vi "总磷总氮测量数据储存.vi"   [LabVIEW 2016, in "斯坦道总磷总氮V2.lvlib"]
types:
  T1 = cluster{"时间标识":timestamp, "测量模式":enum16{"维护数据", "水样测试", "标样核查", "零点核查", "跨度核查", "空白测试", "平行样测试", "加标回收", "空白校准", "标样校准", "初始化（清洗）", "快捷测试"}, "数据标记表":string, "监测值":sgl, "单位":u16, "数据标识":string, "因子编码":u32, "标样参考值":sgl, "F0":sgl, "F1":sgl, "F2":sgl, "F3":sgl, "F4":sgl, "F5":sgl, "F6":sgl, "F7":sgl, "X":sgl, "温度":sgl, "湿度":sgl, "量程标识":string, "SN":string, "跨度值":sgl, "X1":sgl}
  T2 = enum16{"维护数据", "水样测试", "标样核查", "零点核查", "跨度核查", "空白测试", "平行样测试", "加标回收", "空白校准", "标样校准", "初始化（清洗）", "快捷测试"}
  T3 = enum16{"维护数据", "水样测试", "标样核查", "零点核查", "跨度核查", "空白测试", "平行样测试", "加标回收", "空白校准", "标样校准", "初始化（清洗）"}
  T4 = cluster{"系统时间":timestamp, "工作状态":u16, "测量模式":enum16{"待机", "连续模式", "周期模式", "定点模式", "受控模式", "手动模式"}, "告警代码":u16, "故障代码":u16, "日志代码":u16, "软件版本":u16, "F0":sgl, "F1":sgl, "F2":sgl, "F3":sgl, "T":sgl, "H":sgl, "id":u16, "flowid":u16, "量程":u16, "总磷控温温度1":sgl, "营养盐控温温度2":sgl, "ADC":sgl}
  T5 = cluster{"运行模式":enum16{"维护模式", "常规模式", "应急模式", "质控模式"}, "质控频次":enum16{"关闭", "每天", "星期一", "星期二", "星期三", "星期四", "星期五", "星期六", "星期日"}, "空白核查时间":u16, "跨度核查时间":u16, "测量间隔":dbl}
  T6 = cluster{"因子编码":u32, "单位":u16, "标样参考值":sgl, "水样数据时间":timestamp, "水样实测值":sgl, "水样数据标识":string, "标样数据时间":timestamp, "标样实测值":sgl, "标样数据标识":string, "空白数据时间":timestamp, "空白实测值":sgl, "空白数据标识":string, "零点核查数据时间":timestamp, "零点核查实测值":sgl, "零点核查数据标识":string, "跨度核查数据时间":timestamp, "跨度核查实测值":sgl, "跨度核查数据标识":string, "加标回收数据时间":timestamp, "加标回收实测值":sgl, "加标回收数据标识":string, "平行样数据时间":timestamp, "平行样实测值":sgl, "平行样数据标识":string, "F0":sgl, "F1":sgl, "F2":sgl, "F3":sgl, "F4":sgl, "F5":sgl, "F6":sgl, "F7":sgl, "温度":sgl, "湿度":sgl, "X值":sgl, "fidrange":u16}[]
  T7 = cluster{"因子编码":u32, "单位":u16, "标样参考值":sgl, "水样数据时间":timestamp, "水样实测值":sgl, "水样数据标识":string, "标样数据时间":timestamp, "标样实测值":sgl, "标样数据标识":string, "空白数据时间":timestamp, "空白实测值":sgl, "空白数据标识":string, "零点核查数据时间":timestamp, "零点核查实测值":sgl, "零点核查数据标识":string, "跨度核查数据时间":timestamp, "跨度核查实测值":sgl, "跨度核查数据标识":string, "加标回收数据时间":timestamp, "加标回收实测值":sgl, "加标回收数据标识":string, "平行样数据时间":timestamp, "平行样实测值":sgl, "平行样数据标识":string, "F0":sgl, "F1":sgl, "F2":sgl, "F3":sgl, "F4":sgl, "F5":sgl, "F6":sgl, "F7":sgl, "温度":sgl, "湿度":sgl, "X值":sgl, "fidrange":u16}
  T8 = cluster{"总磷跨度值":dbl, "总磷零点标准液浓度":dbl, "总磷跨度标准液浓度":dbl, "总磷标准液标准浓度":dbl, "总氮跨度值":dbl, "总氮零点标准液浓度":dbl, "总氮跨度标准液浓度":dbl, "总氮标准液标准浓度":dbl, "COD跨度值":dbl, "COD零点标准液浓度":dbl, "COD跨度标准液浓度":dbl, "COD标准液标准浓度":dbl, "氨氮跨度值":dbl, "氨氮零点标准液浓度":dbl, "氨氮跨度标准液浓度":dbl, "氨氮标准液标准浓度":dbl, "磷酸盐跨度值":dbl, "磷酸盐零点标准液浓度":dbl, "磷酸盐跨度标准液浓度":dbl, "磷酸盐标准液标准浓度":dbl, "硝氮跨度值":dbl, "硝氮零点标准液浓度":dbl, "硝氮跨度标准液浓度":dbl, "硝氮标准液标准浓度":dbl, "亚硝氮跨度值":dbl, "亚硝氮零点标准液浓度":dbl, "亚硝氮跨度标准液浓度":dbl, "亚硝氮标准液标准浓度":dbl, "硫化物跨度值":dbl, "硫化物零点标准液浓度":dbl, "硫化物跨度标准液浓度":dbl, "硫化物标准液标准浓度":dbl, "硅酸盐跨度值":dbl, "硅酸盐零点标准液浓度":dbl, "硅酸盐跨度标准液浓度":dbl, "硅酸盐标准液标准浓度":dbl}
  T9 = typedef "斯坦道总磷总氮V2.lvlib/关键参数.ctl" = cluster{"测量量程":sgl, "测量检出限":sgl, "测量精度":sgl, "测量间隔":sgl, "消解温度":sgl, "消解时长":sgl, "三项式系数":sgl, "二次多项式系数":sgl, "曲线斜率":sgl, "曲线截距":sgl, "线性相关系数":sgl, "空白校准时间":timestamp, "标样校准时间":timestamp, "测量信号值":sgl, "稀释倍数":sgl, "空白标定系数":sgl, "量程系数":sgl}
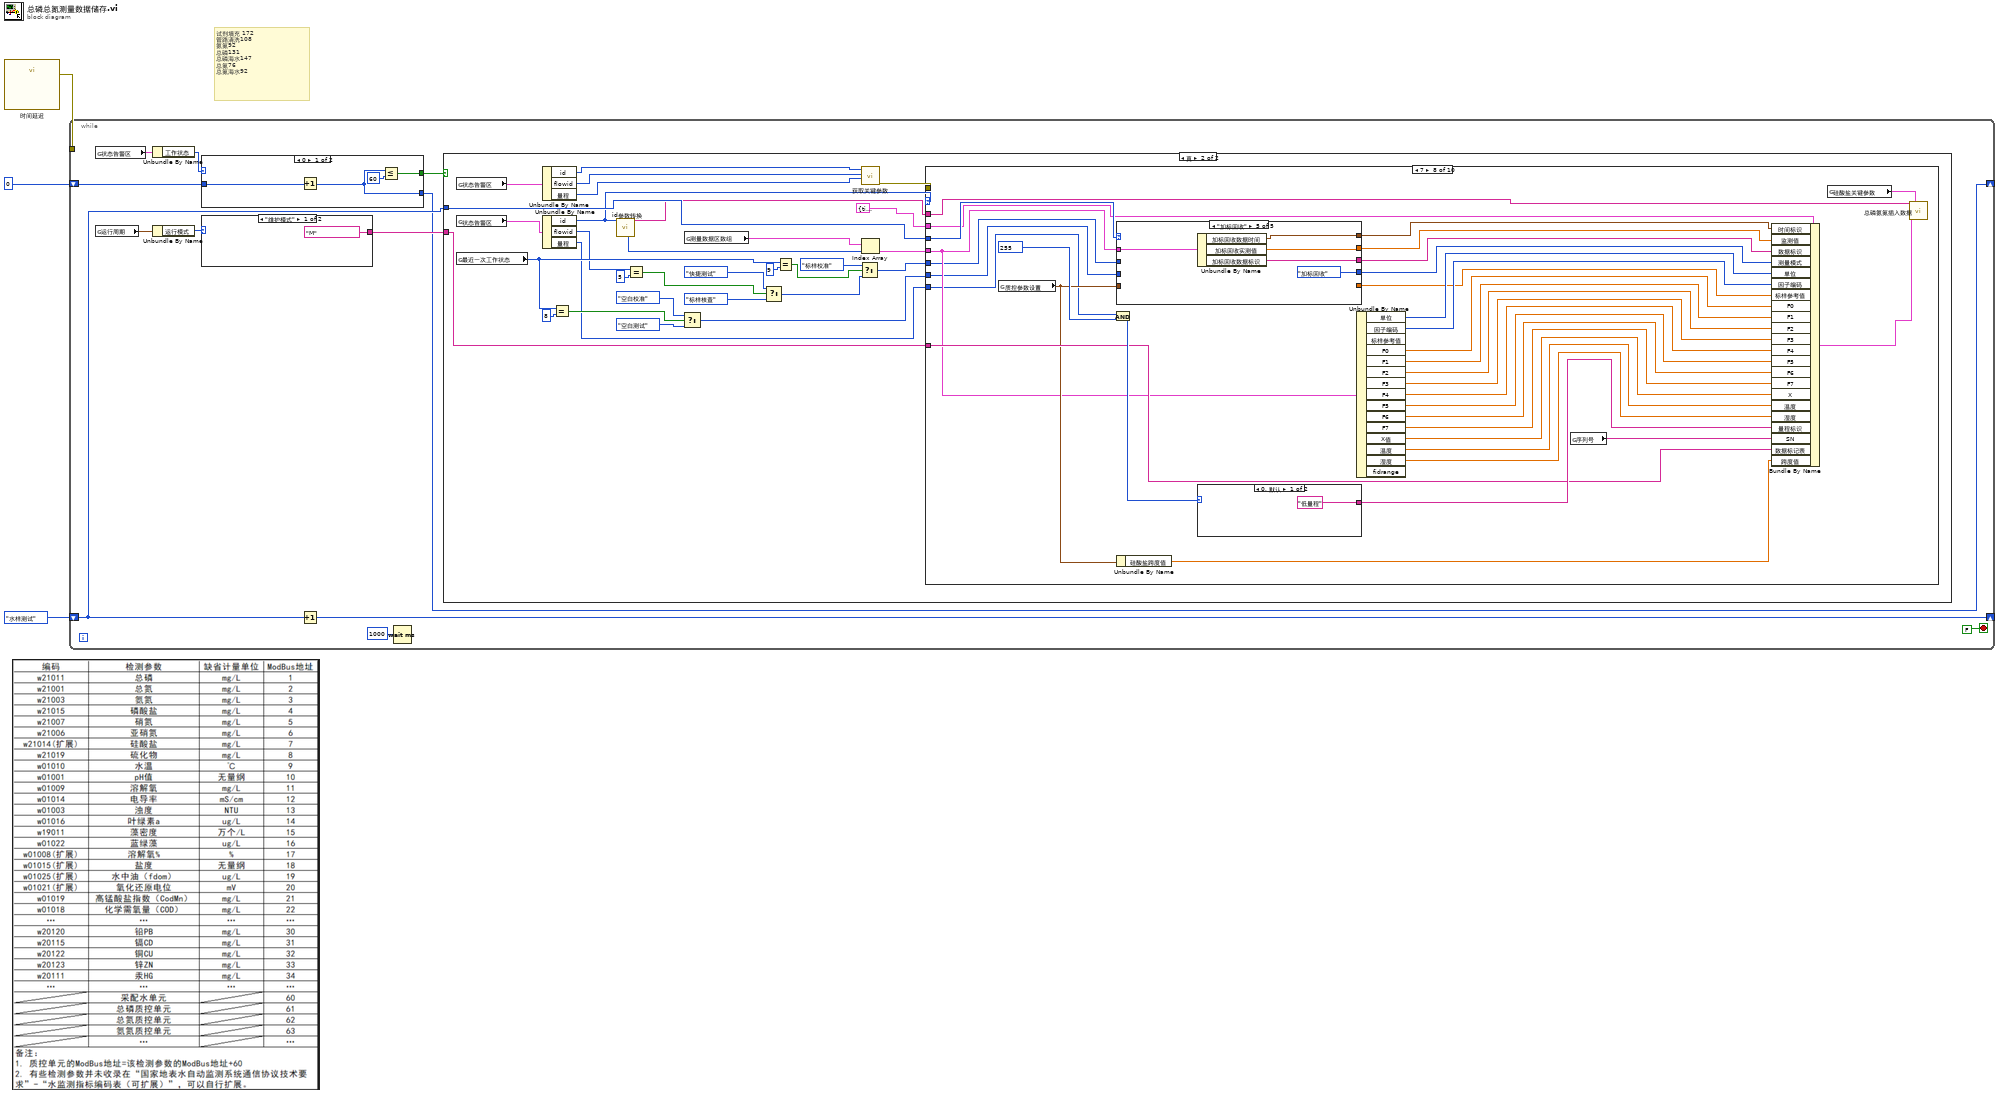
[diagram p0: block diagram]
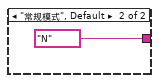
[diagram p3: hidden frame]
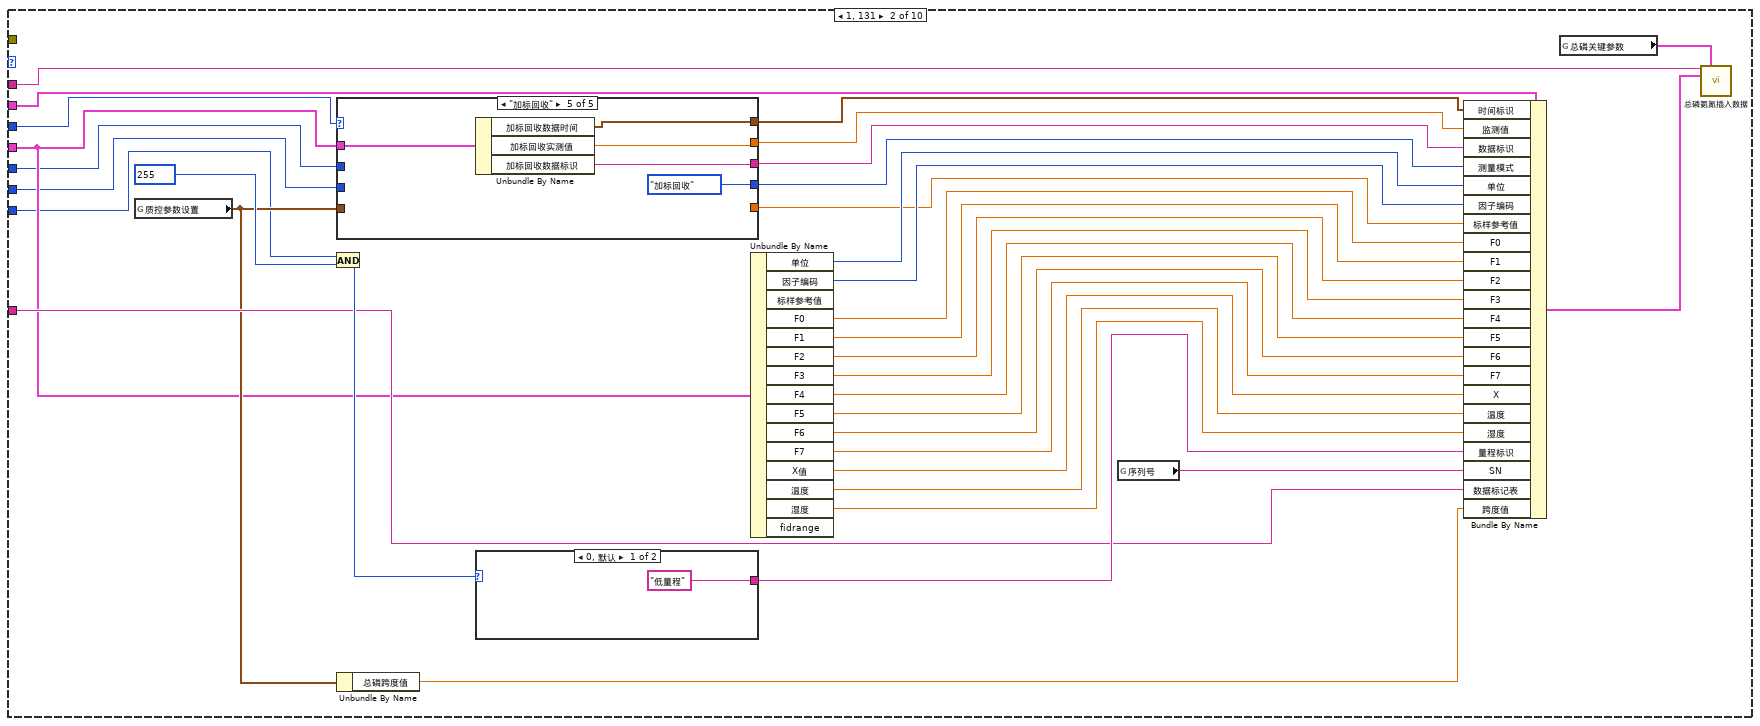
[diagram p6: hidden frame]
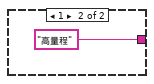
[diagram p7: hidden frame]
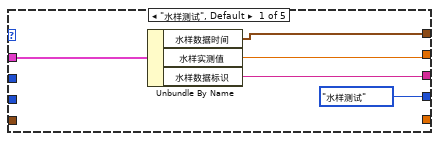
[diagram p8: hidden frame]
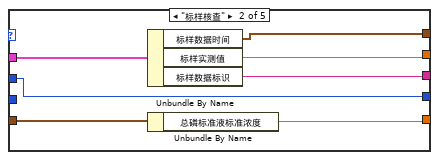
[diagram p9: hidden frame]
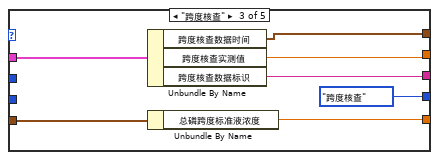
[diagram p10: hidden frame]
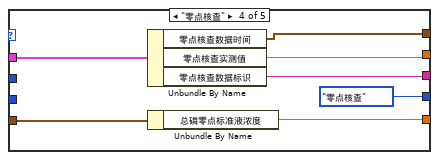
[diagram p11: hidden frame]
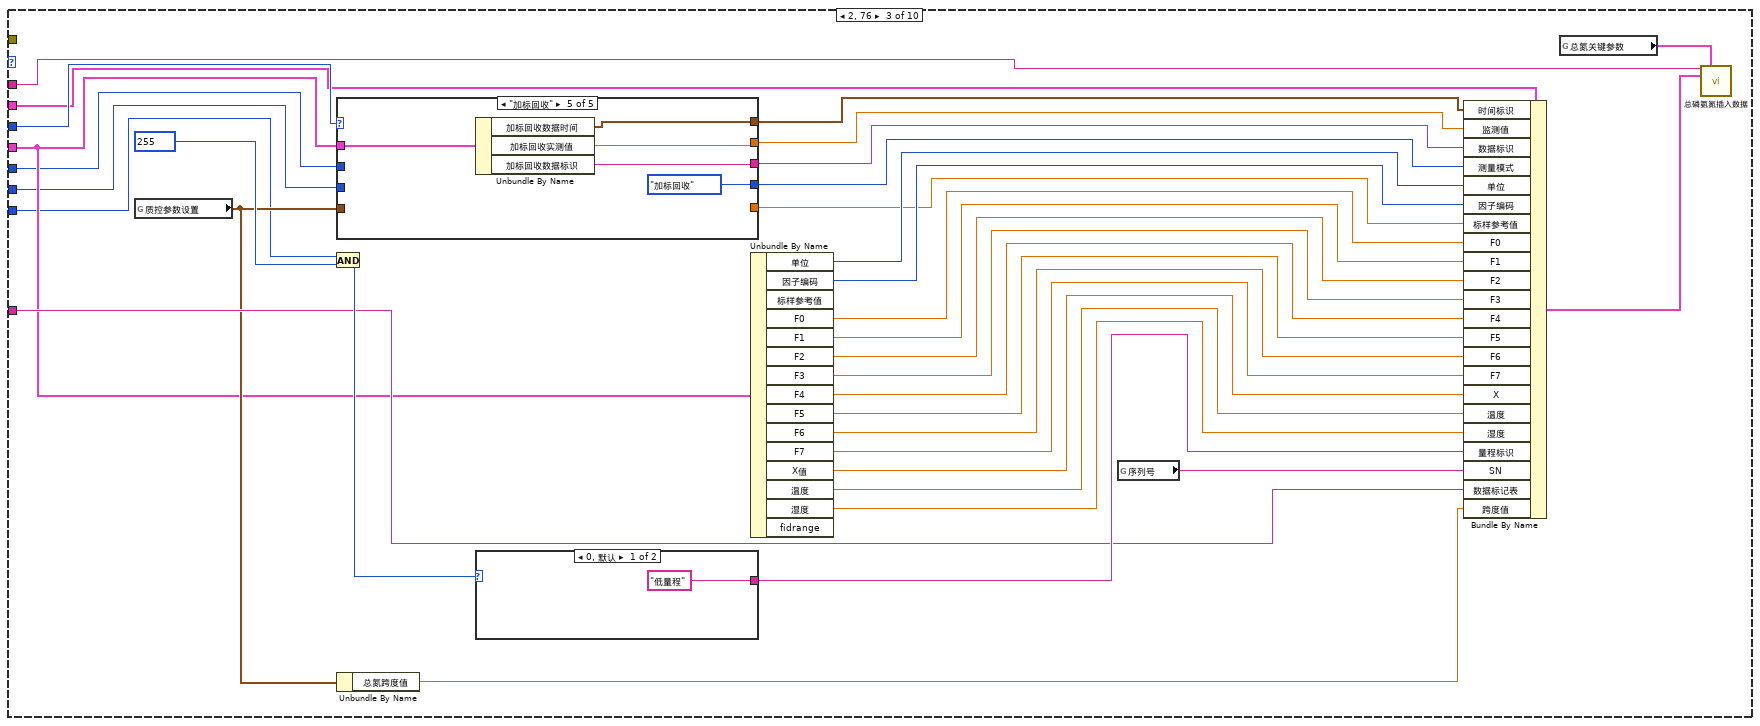
[diagram p12: hidden frame]
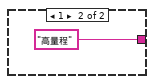
[diagram p13: hidden frame]
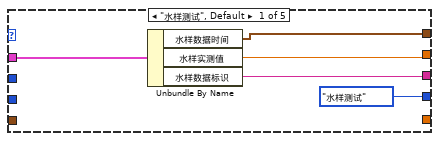
[diagram p14: hidden frame]
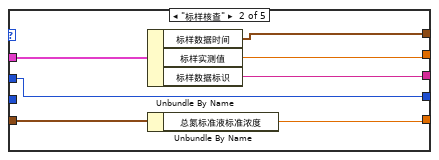
[diagram p15: hidden frame]
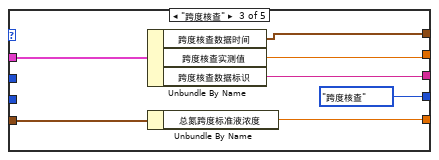
[diagram p16: hidden frame]
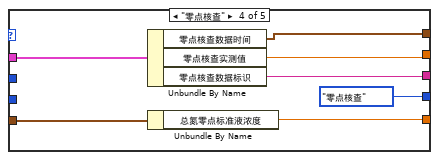
[diagram p17: hidden frame]
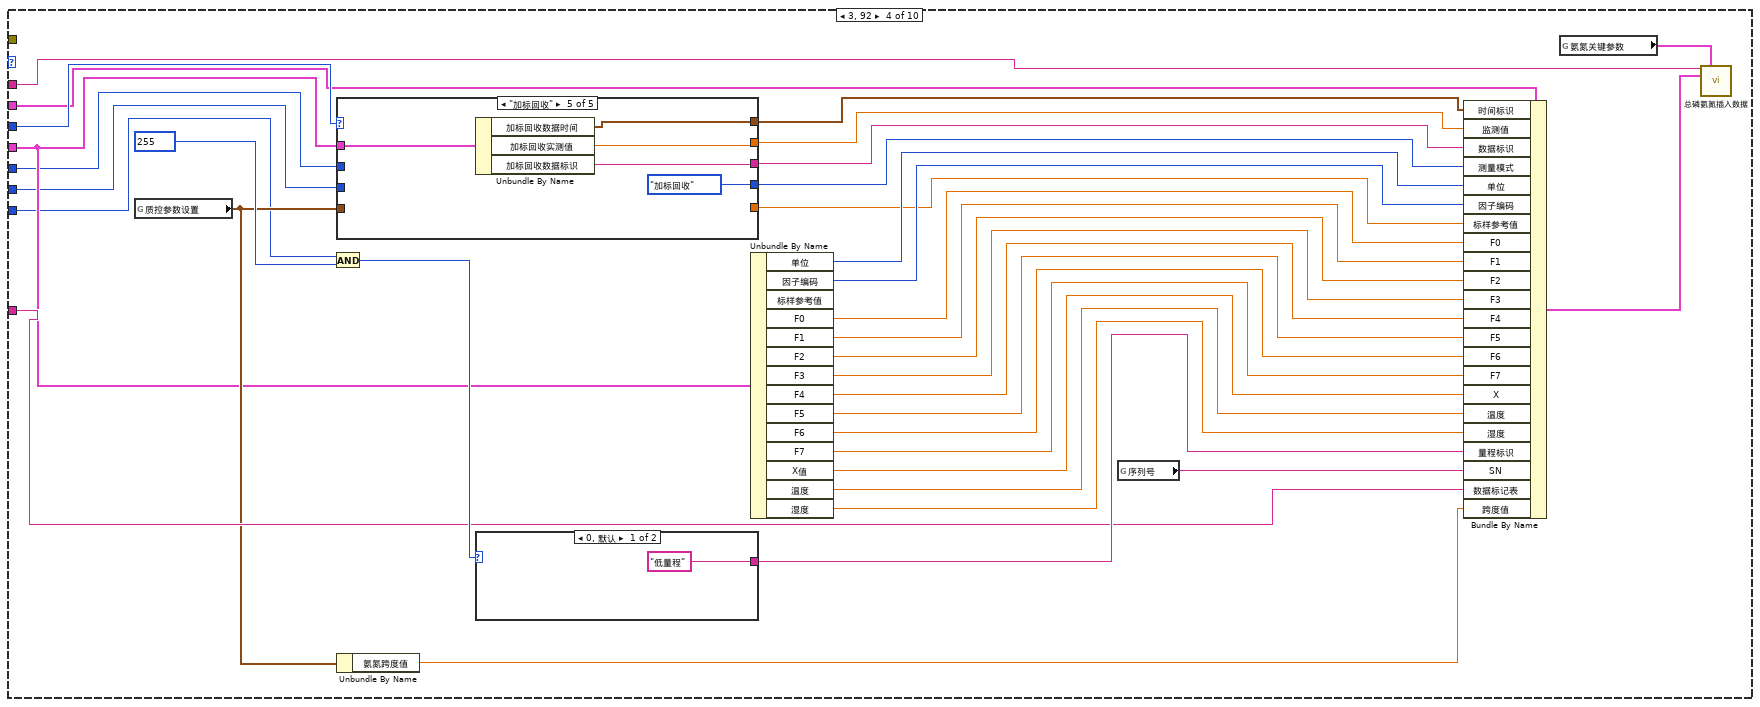
[diagram p18: hidden frame]
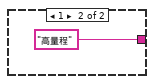
[diagram p19: hidden frame]
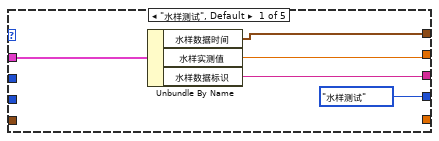
[diagram p20: hidden frame]
diagram:
  # "试剂填充 172 \n管路清洗108\n氨氮92\n总磷131\n总磷海水147\n总氮76\n总氮海水92"
  n1 = call "时间延迟"() -> ("error out"=w1:errorcluster)  [unwired: 11 in]
  n2 = while {
    shift-right: [w13] -> _
    shift-left: enum16{"水样测试", "标样核查", "跨度核查", "零点核查", "加标回收"}."水样测试" ("测量模式") -> [w12]
    shift-right: [w6] -> _
    shift-left: u32 0 ("等待时间（毫秒）") -> [w7]
    tunnel: w1 -> [_]
    stop <- FALSE stop-if-true
    n3 = global read "VAR总磷总氮全局变量.vi" "状态告警区"() -> (w9:T4)
    n4 = global read "总磷总氮断电保存全局变量.vi" "运行周期"() -> (w11:T5)
    n5 = Unbundle By Name(w9) -> ("工作状态"=w8:u16)
    n6 = Unbundle By Name(w11) -> ("运行模式"=w10:enum16{"维护模式", "常规模式", "应急模式", "质控模式"})
    n7 = case shown="0" w8 {
      tunnel: w7 -> [w19 _]
      tunnel: [w18 _] -> w6
      tunnel: [w16 _] -> w5
      frame 0 {
        n8 = Increment(x=w19) -> (x+1=w18:u32)
        n9 = Less Or Equal?(x=w18, y=u32 60) -> (x <= y?=w16:bool)
      }
      frame 1, Default {
      }
    }
    n10 = case shown="\"维护模式\"" w10 {
      tunnel: ["M" ("数据标记表") "N" ("数据标记表")] -> w14
      frame "维护模式" {
      }
      frame "常规模式", Default {
      }
    }
    n11 = Increment(x=w12) -> (x+1=w13:enum16{"水样测试", "标样核查", "跨度核查", "零点核查", "加标回收"})
    n12 = Wait (ms)(milliseconds to wait=u32 1000 ("等待时间（毫秒）")) -> ()  [unwired: 1 out]
    n13 = case shown="真" w5 {
      tunnel: w14 -> [_ w52]
      tunnel: w12 -> [_ w51]
      frame False {
      }
      frame True {
        n14 = global read "VAR总磷总氮全局变量.vi" "状态告警区"() -> (w27:T4)
        n15 = global read "VAR总磷总氮全局变量.vi" "状态告警区"() -> (w50:T4)
        n16 = global read "VAR总磷总氮全局变量.vi" "最近一次工作状态"() -> (w37:u16)
        n17 = Unbundle By Name(w27) -> ("id"=w26:u16, "flowid"=w25:u16, "量程"=w24:u16)
        n18 = Unbundle By Name(w50) -> ("id"=w47:u16, "flowid"=w34:u16, "量程"=w28:u16)
        n19 = Equal?(x=w37, y=u16 8) -> (x = y?=w43:bool)
        n20 = call "id参数转换.vi"("id"=w47) -> ("table输出"=w46:string, "数组资源索引"=w45:i32)  [unwired: 9 in]
        n21 = Equal?(x=w34, y=u16 5) -> (x = y?=w32:bool)
        n22 = Select(t=T2."空白校准" ("测量模式"), s=w43, f=T2."空白测试" ("测量模式")) -> (s? t:f=w36:T2)
        n23 = global read "VAR总磷总氮全局变量.vi" "测量数据区数组"() -> (w49:T6)
        n24 = Select(t=T2."快捷测试" ("测量模式"), s=w32, f=T2."标样核查" ("测量模式")) -> (s? t:f=w29:T2)
        n25 = Equal?(x=w37, y=u16 9) -> (x = y?=w39:bool)
        n26 = Select(t=T2."标样校准" ("测量模式"), s=w39, f=w29) -> (s? t:f=w35:T2)
        n27 = call "获取关键参数.vi"("量程"=w24, "flowid"=w25, "id"=w26) -> ("error out"=w23:errorcluster)  [unwired: 8 in]
        n28 = Index Array(array=w49, index=w45) -> (element=w48:T7)
        n29 = case shown="7" w47 {
          tunnel: w52 -> [_ w63 w130 w198 w265 w332 w399 w466 w533 w600]
          tunnel: w51 -> [_ w70 w140 w207 w274 w341 w408 w475 w542 w609]
          tunnel: T1 {"时间标识"=timestamp(0 s since 1904-01-01), "测量模式"=enum."水样测试", "数据标记表"="N", "监测值"=0.0, "单位"=0, "数据标识"="", "因子编码"=0, "标样参考值"=0.0, "F0"=0.0, "F1"=0.0, "F2"=0.0, "F3"=0.0, "F4"=0.0, "F5"=0.0, "F6"=0.0, "F7"=0.0, "X"=0.0, "温度"=0.0, "湿度"=0.0, "量程标识"="", "SN"="", "跨度值"=0.0, "X1"=0.0} ("data") -> [_ w61 w128 w196 w263 w330 w397 w464 w531 w598]
          tunnel: w48 -> [_ w58 w125 w193 w260 w327 w394 w461 w528 w594]
          tunnel: w46 -> [_ w57 w124 w191 w258 w325 w392 w460 w526 w593]
          tunnel: w36 -> [_ w56 w123 w189 w257 w324 w391 w458 w525 w592]
          tunnel: w35 -> [_ w55 w122 w190 w256 w323 w390 w459 w524 w591]
          tunnel: w28 -> [_ w53 w120 w187 w254 w321 w388 w456 w522 w589]
          tunnel: w23 -> [_ _ _ _ _ _ _ _ _ _]
          frame Default {
          }
          frame 1, 131 {
            n30 = global read "总磷总氮断电保存全局变量.vi" "质控参数设置"() -> (w60:T8)
            n31 = And(x=w53, y=u16 255) -> (x .and. y?=w67:u16)
            n32 = case shown="\"加标回收\"" w70 {
              tunnel: w58 -> [w93 w100 w107 w114 w119]
              tunnel: [w92 w99 w106 w113 w118] -> w71
              tunnel: [w91 w98 w105 w112 w117] -> w72
              tunnel: [w90 w97 w104 w111 w116] -> w73
              tunnel: [T3."水样测试" ("测量模式") w94 T3."跨度核查" ("测量模式") T3."零点核查" ("测量模式") T3."加标回收" ("测量模式")] -> w62
              tunnel: w60 -> [_ w96 w102 w109 _]
              tunnel: [_ w95 w101 w108 _] -> w69
              tunnel: w56 -> [_ _ _ _ _]
              tunnel: w55 -> [_ w94 _ _ _]
              frame "水样测试", Default {
                n33 = Unbundle By Name(w93) -> ("水样数据时间"=w92:timestamp, "水样实测值"=w91:sgl, "水样数据标识"=w90:string)
              }
              frame "标样核查" {
                n34 = Unbundle By Name(w100) -> ("标样数据时间"=w99:timestamp, "标样实测值"=w98:sgl, "标样数据标识"=w97:string)
                n35 = Unbundle By Name(w96) -> ("总磷标准液标准浓度"=w95:dbl)
              }
              frame "跨度核查" {
                n36 = Unbundle By Name(w107) -> ("跨度核查数据时间"=w106:timestamp, "跨度核查实测值"=w105:sgl, "跨度核查数据标识"=w104:string)
                n37 = Unbundle By Name(w102) -> ("总磷跨度标准液浓度"=w101:dbl)
              }
              frame "零点核查" {
                n38 = Unbundle By Name(w114) -> ("零点核查数据时间"=w113:timestamp, "零点核查实测值"=w112:sgl, "零点核查数据标识"=w111:string)
                n39 = Unbundle By Name(w109) -> ("总磷零点标准液浓度"=w108:dbl)
              }
              frame "加标回收" {
                n40 = Unbundle By Name(w119) -> ("加标回收数据时间"=w118:timestamp, "加标回收实测值"=w117:sgl, "加标回收数据标识"=w116:string)
              }
            }
            n41 = Unbundle By Name(w60) -> ("总磷跨度值"=w59:dbl)
            n42 = case shown="0, 默认" w67 {
              tunnel: ["低量程" ("格式字符串") "高量程" ("格式字符串")] -> w66
              frame 0, Default {
              }
              frame 1 {
              }
            }
            n43 = Unbundle By Name(w58) -> ("单位"=w86:u16, "因子编码"=w85:u32, "F0"=w84:sgl, "F1"=w83:sgl, "F2"=w82:sgl, "F3"=w81:sgl, "F4"=w80:sgl, "F5"=w79:sgl, "F6"=w78:sgl, "F7"=w77:sgl, "X值"=w76:sgl, "温度"=w75:sgl, "湿度"=w74:sgl)  [unwired: 2 out]
            n44 = global read "VAR总磷总氮全局变量.vi" "序列号"() -> (w64:string)
            n45 = Bundle By Name(cluster=w61, "时间标识"=w71, "监测值"=w72, "数据标识"=w73, "测量模式"=w62, "单位"=w86, "因子编码"=w85, "标样参考值"=w69, "F0"=w84, "F1"=w83, "F2"=w82, "F3"=w81, "F4"=w80, "F5"=w79, "F6"=w78, "F7"=w77, "X"=w76, "温度"=w75, "湿度"=w74, "量程标识"=w66, "SN"=w64, "数据标记表"=w63, "跨度值"=w59) -> (w65:T1)
            n46 = global read "VAR总磷总氮全局变量.vi" "总磷关键参数"() -> (w54:T9)
            n47 = call "总磷氨氮插入数据.vi"("table"=w57, "关键参数"=w54, "data"=w65) -> ()  [unwired: 12 in, 1 out]
          }
          frame 2, 76 {
            n48 = global read "总磷总氮断电保存全局变量.vi" "质控参数设置"() -> (w127:T8)
            n49 = And(x=w120, y=u16 255) -> (x .and. y?=w134:u16)
            n50 = case shown="\"加标回收\"" w140 {
              tunnel: w125 -> [w160 w167 w174 w181 w186]
              tunnel: [w159 w166 w173 w180 w185] -> w139
              tunnel: [w158 w165 w172 w179 w184] -> w138
              tunnel: [w157 w164 w171 w178 w183] -> w137
              tunnel: [T3."水样测试" ("测量模式") w161 T3."跨度核查" ("测量模式") T3."零点核查" ("测量模式") T3."加标回收" ("测量模式")] -> w129
              tunnel: w127 -> [_ w163 w169 w176 _]
              tunnel: [_ w162 w168 w175 _] -> w136
              tunnel: w123 -> [_ _ _ _ _]
              tunnel: w122 -> [_ w161 _ _ _]
              frame "水样测试", Default {
                n51 = Unbundle By Name(w160) -> ("水样数据时间"=w159:timestamp, "水样实测值"=w158:sgl, "水样数据标识"=w157:string)
              }
              frame "标样核查" {
                n52 = Unbundle By Name(w167) -> ("标样数据时间"=w166:timestamp, "标样实测值"=w165:sgl, "标样数据标识"=w164:string)
                n53 = Unbundle By Name(w163) -> ("总氮标准液标准浓度"=w162:dbl)
              }
              frame "跨度核查" {
                n54 = Unbundle By Name(w174) -> ("跨度核查数据时间"=w173:timestamp, "跨度核查实测值"=w172:sgl, "跨度核查数据标识"=w171:string)
                n55 = Unbundle By Name(w169) -> ("总氮跨度标准液浓度"=w168:dbl)
              }
              frame "零点核查" {
                n56 = Unbundle By Name(w181) -> ("零点核查数据时间"=w180:timestamp, "零点核查实测值"=w179:sgl, "零点核查数据标识"=w178:string)
                n57 = Unbundle By Name(w176) -> ("总氮零点标准液浓度"=w175:dbl)
              }
              frame "加标回收" {
                n58 = Unbundle By Name(w186) -> ("加标回收数据时间"=w185:timestamp, "加标回收实测值"=w184:sgl, "加标回收数据标识"=w183:string)
              }
            }
            n59 = Unbundle By Name(w127) -> ("总氮跨度值"=w126:dbl)
            n60 = case shown="0, 默认" w134 {
              tunnel: ["低量程" ("格式字符串") "高量程" ("格式字符串")] -> w133
              frame 0, Default {
              }
              frame 1 {
              }
            }
            n61 = Unbundle By Name(w125) -> ("单位"=w153:u16, "因子编码"=w152:u32, "F0"=w151:sgl, "F1"=w150:sgl, "F2"=w149:sgl, "F3"=w148:sgl, "F4"=w147:sgl, "F5"=w146:sgl, "F6"=w145:sgl, "F7"=w144:sgl, "X值"=w143:sgl, "温度"=w142:sgl, "湿度"=w141:sgl)  [unwired: 2 out]
            n62 = global read "VAR总磷总氮全局变量.vi" "序列号"() -> (w131:string)
            n63 = Bundle By Name(cluster=w128, "时间标识"=w139, "监测值"=w138, "数据标识"=w137, "测量模式"=w129, "单位"=w153, "因子编码"=w152, "标样参考值"=w136, "F0"=w151, "F1"=w150, "F2"=w149, "F3"=w148, "F4"=w147, "F5"=w146, "F6"=w145, "F7"=w144, "X"=w143, "温度"=w142, "湿度"=w141, "量程标识"=w133, "SN"=w131, "数据标记表"=w130, "跨度值"=w126) -> (w132:T1)
            n64 = global read "VAR总磷总氮全局变量.vi" "总氮关键参数"() -> (w121:T9)
            n65 = call "总磷氨氮插入数据.vi"("table"=w124, "关键参数"=w121, "data"=w132) -> ()  [unwired: 12 in, 1 out]
          }
          frame 3, 92 {
            n66 = global read "总磷总氮断电保存全局变量.vi" "质控参数设置"() -> (w195:T8)
            n67 = And(x=w187, y=u16 255) -> (x .and. y?=w201:u16)
            n68 = case shown="\"加标回收\"" w207 {
              tunnel: w193 -> [w227 w234 w241 w248 w253]
              tunnel: [w226 w233 w240 w247 w252] -> w206
              tunnel: [w225 w232 w239 w246 w251] -> w205
              tunnel: [w224 w231 w238 w245 w250] -> w204
              tunnel: [T3."水样测试" ("测量模式") w228 T3."跨度核查" ("测量模式") T3."零点核查" ("测量模式") T3."加标回收" ("测量模式")] -> w197
              tunnel: w195 -> [_ w230 w236 w243 _]
              tunnel: [_ w229 w235 w242 _] -> w203
              tunnel: w190 -> [_ w228 _ _ _]
              tunnel: w189 -> [_ _ _ _ _]
              frame "水样测试", Default {
                n69 = Unbundle By Name(w227) -> ("水样数据时间"=w226:timestamp, "水样实测值"=w225:sgl, "水样数据标识"=w224:string)
              }
              frame "标样核查" {
                n70 = Unbundle By Name(w234) -> ("标样数据时间"=w233:timestamp, "标样实测值"=w232:sgl, "标样数据标识"=w231:string)
                n71 = Unbundle By Name(w230) -> ("氨氮标准液标准浓度"=w229:dbl)
              }
              frame "跨度核查" {
                n72 = Unbundle By Name(w241) -> ("跨度核查数据时间"=w240:timestamp, "跨度核查实测值"=w239:sgl, "跨度核查数据标识"=w238:string)
                n73 = Unbundle By Name(w236) -> ("氨氮跨度标准液浓度"=w235:dbl)
              }
              frame "零点核查" {
                n74 = Unbundle By Name(w248) -> ("零点核查数据时间"=w247:timestamp, "零点核查实测值"=w246:sgl, "零点核查数据标识"=w245:string)
                n75 = Unbundle By Name(w243) -> ("氨氮零点标准液浓度"=w242:dbl)
              }
              frame "加标回收" {
                n76 = Unbundle By Name(w253) -> ("加标回收数据时间"=w252:timestamp, "加标回收实测值"=w251:sgl, "加标回收数据标识"=w250:string)
              }
            }
            n77 = Unbundle By Name(w195) -> ("氨氮跨度值"=w194:dbl)
            n78 = case shown="0, 默认" w201 {
              tunnel: ["低量程" ("格式字符串") "高量程" ("格式字符串")] -> w200
              frame 0, Default {
              }
              frame 1 {
              }
            }
            n79 = Unbundle By Name(w193) -> ("单位"=w220:u16, "因子编码"=w219:u32, "F0"=w218:sgl, "F1"=w217:sgl, "F2"=w216:sgl, "F3"=w215:sgl, "F4"=w214:sgl, "F5"=w213:sgl, "F6"=w212:sgl, "F7"=w211:sgl, "X值"=w210:sgl, "温度"=w209:sgl, "湿度"=w208:sgl)  [unwired: 1 out]
            n80 = global read "VAR总磷总氮全局变量.vi" "序列号"() -> (w199:string)
            n81 = Bundle By Name(cluster=w196, "时间标识"=w206, "监测值"=w205, "数据标识"=w204, "测量模式"=w197, "单位"=w220, "因子编码"=w219, "标样参考值"=w203, "F0"=w218, "F1"=w217, "F2"=w216, "F3"=w215, "F4"=w214, "F5"=w213, "F6"=w212, "F7"=w211, "X"=w210, "温度"=w209, "湿度"=w208, "量程标识"=w200, "SN"=w199, "数据标记表"=w198, "跨度值"=w194) -> (w192:T1)
            n82 = global read "VAR总磷总氮全局变量.vi" "氨氮关键参数"() -> (w188:T9)
            n83 = call "总磷氨氮插入数据.vi"("table"=w191, "关键参数"=w188, "data"=w192) -> ()  [unwired: 12 in, 1 out]
          }
          frame 4 {
            n84 = global read "总磷总氮断电保存全局变量.vi" "质控参数设置"() -> (w262:T8)
            n85 = And(x=w254, y=u16 255) -> (x .and. y?=w268:u16)
            n86 = case shown="\"加标回收\"" w274 {
              tunnel: w260 -> [w294 w301 w308 w315 w320]
              tunnel: [w293 w300 w307 w314 w319] -> w273
              tunnel: [w292 w299 w306 w313 w318] -> w272
              tunnel: [w291 w298 w305 w312 w317] -> w271
              tunnel: [T3."水样测试" ("测量模式") w295 T3."跨度核查" ("测量模式") T3."零点核查" ("测量模式") T3."加标回收" ("测量模式")] -> w264
              tunnel: w262 -> [_ w297 w303 w310 _]
              tunnel: [_ w296 w302 w309 _] -> w270
              tunnel: w257 -> [_ _ _ _ _]
              tunnel: w256 -> [_ w295 _ _ _]
              frame "水样测试", Default {
                n87 = Unbundle By Name(w294) -> ("水样数据时间"=w293:timestamp, "水样实测值"=w292:sgl, "水样数据标识"=w291:string)
              }
              frame "标样核查" {
                n88 = Unbundle By Name(w301) -> ("标样数据时间"=w300:timestamp, "标样实测值"=w299:sgl, "标样数据标识"=w298:string)
                n89 = Unbundle By Name(w297) -> ("磷酸盐标准液标准浓度"=w296:dbl)
              }
              frame "跨度核查" {
                n90 = Unbundle By Name(w308) -> ("跨度核查数据时间"=w307:timestamp, "跨度核查实测值"=w306:sgl, "跨度核查数据标识"=w305:string)
                n91 = Unbundle By Name(w303) -> ("磷酸盐跨度标准液浓度"=w302:dbl)
              }
              frame "零点核查" {
                n92 = Unbundle By Name(w315) -> ("零点核查数据时间"=w314:timestamp, "零点核查实测值"=w313:sgl, "零点核查数据标识"=w312:string)
                n93 = Unbundle By Name(w310) -> ("磷酸盐零点标准液浓度"=w309:dbl)
              }
              frame "加标回收" {
                n94 = Unbundle By Name(w320) -> ("加标回收数据时间"=w319:timestamp, "加标回收实测值"=w318:sgl, "加标回收数据标识"=w317:string)
              }
            }
            n95 = Unbundle By Name(w262) -> ("磷酸盐跨度值"=w261:dbl)
            n96 = case shown="0, 默认" w268 {
              tunnel: ["低量程" ("格式字符串") "高量程" ("格式字符串")] -> w267
              frame 0, Default {
              }
              frame 1 {
              }
            }
            n97 = Unbundle By Name(w260) -> ("单位"=w287:u16, "因子编码"=w286:u32, "F0"=w285:sgl, "F1"=w284:sgl, "F2"=w283:sgl, "F3"=w282:sgl, "F4"=w281:sgl, "F5"=w280:sgl, "F6"=w279:sgl, "F7"=w278:sgl, "X值"=w277:sgl, "温度"=w276:sgl, "湿度"=w275:sgl)  [unwired: 2 out]
            n98 = global read "VAR总磷总氮全局变量.vi" "序列号"() -> (w266:string)
            n99 = Bundle By Name(cluster=w263, "时间标识"=w273, "监测值"=w272, "数据标识"=w271, "测量模式"=w264, "单位"=w287, "因子编码"=w286, "标样参考值"=w270, "F0"=w285, "F1"=w284, "F2"=w283, "F3"=w282, "F4"=w281, "F5"=w280, "F6"=w279, "F7"=w278, "X"=w277, "温度"=w276, "湿度"=w275, "量程标识"=w267, "SN"=w266, "数据标记表"=w265, "跨度值"=w261) -> (w259:T1)
            n100 = global read "VAR总磷总氮全局变量.vi" "磷酸盐关键参数"() -> (w255:T9)
            n101 = call "总磷氨氮插入数据.vi"("table"=w258, "关键参数"=w255, "data"=w259) -> ()  [unwired: 12 in, 1 out]
          }
          frame 5 {
            n102 = global read "总磷总氮断电保存全局变量.vi" "质控参数设置"() -> (w329:T8)
            n103 = And(x=w321, y=u16 255) -> (x .and. y?=w335:u16)
            n104 = case shown="\"加标回收\"" w341 {
              tunnel: w327 -> [w361 w368 w375 w382 w387]
              tunnel: [w360 w367 w374 w381 w386] -> w340
              tunnel: [w359 w366 w373 w380 w385] -> w339
              tunnel: [w358 w365 w372 w379 w384] -> w338
              tunnel: [T3."水样测试" ("测量模式") w362 T3."跨度核查" ("测量模式") T3."零点核查" ("测量模式") T3."加标回收" ("测量模式")] -> w331
              tunnel: w329 -> [_ w364 w370 w377 _]
              tunnel: [_ w363 w369 w376 _] -> w337
              tunnel: w324 -> [_ _ _ _ _]
              tunnel: w323 -> [_ w362 _ _ _]
              frame "水样测试", Default {
                n105 = Unbundle By Name(w361) -> ("水样数据时间"=w360:timestamp, "水样实测值"=w359:sgl, "水样数据标识"=w358:string)
              }
              frame "标样核查" {
                n106 = Unbundle By Name(w368) -> ("标样数据时间"=w367:timestamp, "标样实测值"=w366:sgl, "标样数据标识"=w365:string)
                n107 = Unbundle By Name(w364) -> ("硝氮标准液标准浓度"=w363:dbl)
              }
              frame "跨度核查" {
                n108 = Unbundle By Name(w375) -> ("跨度核查数据时间"=w374:timestamp, "跨度核查实测值"=w373:sgl, "跨度核查数据标识"=w372:string)
                n109 = Unbundle By Name(w370) -> ("硝氮跨度标准液浓度"=w369:dbl)
              }
              frame "零点核查" {
                n110 = Unbundle By Name(w382) -> ("零点核查数据时间"=w381:timestamp, "零点核查实测值"=w380:sgl, "零点核查数据标识"=w379:string)
                n111 = Unbundle By Name(w377) -> ("硝氮零点标准液浓度"=w376:dbl)
              }
              frame "加标回收" {
                n112 = Unbundle By Name(w387) -> ("加标回收数据时间"=w386:timestamp, "加标回收实测值"=w385:sgl, "加标回收数据标识"=w384:string)
              }
            }
            n113 = Unbundle By Name(w329) -> ("硝氮跨度值"=w328:dbl)
            n114 = case shown="0, 默认" w335 {
              tunnel: ["低量程" ("格式字符串") "高量程" ("格式字符串")] -> w334
              frame 0, Default {
              }
              frame 1 {
              }
            }
            n115 = Unbundle By Name(w327) -> ("单位"=w354:u16, "因子编码"=w353:u32, "F0"=w352:sgl, "F1"=w351:sgl, "F2"=w350:sgl, "F3"=w349:sgl, "F4"=w348:sgl, "F5"=w347:sgl, "F6"=w346:sgl, "F7"=w345:sgl, "X值"=w344:sgl, "温度"=w343:sgl, "湿度"=w342:sgl)  [unwired: 2 out]
            n116 = global read "VAR总磷总氮全局变量.vi" "序列号"() -> (w333:string)
            n117 = Bundle By Name(cluster=w330, "时间标识"=w340, "监测值"=w339, "数据标识"=w338, "测量模式"=w331, "单位"=w354, "因子编码"=w353, "标样参考值"=w337, "F0"=w352, "F1"=w351, "F2"=w350, "F3"=w349, "F4"=w348, "F5"=w347, "F6"=w346, "F7"=w345, "X"=w344, "温度"=w343, "湿度"=w342, "量程标识"=w334, "SN"=w333, "数据标记表"=w332, "跨度值"=w328) -> (w326:T1)
            n118 = global read "VAR总磷总氮全局变量.vi" "硝氮关键参数"() -> (w322:T9)
            n119 = call "总磷氨氮插入数据.vi"("table"=w325, "关键参数"=w322, "data"=w326) -> ()  [unwired: 12 in, 1 out]
          }
          frame 6 {
            n120 = global read "总磷总氮断电保存全局变量.vi" "质控参数设置"() -> (w396:T8)
            n121 = And(x=w388, y=u16 255) -> (x .and. y?=w402:u16)
            n122 = case shown="\"加标回收\"" w408 {
              tunnel: w394 -> [w428 w435 w442 w449 w454]
              tunnel: [w427 w434 w441 w448 w453] -> w407
              tunnel: [w426 w433 w440 w447 w452] -> w406
              tunnel: [w425 w432 w439 w446 w451] -> w405
              tunnel: [T3."水样测试" ("测量模式") w429 T3."跨度核查" ("测量模式") T3."零点核查" ("测量模式") T3."加标回收" ("测量模式")] -> w398
              tunnel: w396 -> [_ w431 w437 w444 _]
              tunnel: [_ w430 w436 w443 _] -> w404
              tunnel: w391 -> [_ _ _ _ _]
              tunnel: w390 -> [_ w429 _ _ _]
              frame "水样测试", Default {
                n123 = Unbundle By Name(w428) -> ("水样数据时间"=w427:timestamp, "水样实测值"=w426:sgl, "水样数据标识"=w425:string)
              }
              frame "标样核查" {
                n124 = Unbundle By Name(w435) -> ("标样数据时间"=w434:timestamp, "标样实测值"=w433:sgl, "标样数据标识"=w432:string)
                n125 = Unbundle By Name(w431) -> ("亚硝氮标准液标准浓度"=w430:dbl)
              }
              frame "跨度核查" {
                n126 = Unbundle By Name(w442) -> ("跨度核查数据时间"=w441:timestamp, "跨度核查实测值"=w440:sgl, "跨度核查数据标识"=w439:string)
                n127 = Unbundle By Name(w437) -> ("亚硝氮跨度标准液浓度"=w436:dbl)
              }
              frame "零点核查" {
                n128 = Unbundle By Name(w449) -> ("零点核查数据时间"=w448:timestamp, "零点核查实测值"=w447:sgl, "零点核查数据标识"=w446:string)
                n129 = Unbundle By Name(w444) -> ("亚硝氮零点标准液浓度"=w443:dbl)
              }
              frame "加标回收" {
                n130 = Unbundle By Name(w454) -> ("加标回收数据时间"=w453:timestamp, "加标回收实测值"=w452:sgl, "加标回收数据标识"=w451:string)
              }
            }
            n131 = Unbundle By Name(w396) -> ("亚硝氮跨度值"=w395:dbl)
            n132 = case shown="0, 默认" w402 {
              tunnel: ["低量程" ("格式字符串") "高量程" ("格式字符串")] -> w401
              frame 0, Default {
              }
              frame 1 {
              }
            }
            n133 = Unbundle By Name(w394) -> ("单位"=w421:u16, "因子编码"=w420:u32, "F0"=w419:sgl, "F1"=w418:sgl, "F2"=w417:sgl, "F3"=w416:sgl, "F4"=w415:sgl, "F5"=w414:sgl, "F6"=w413:sgl, "F7"=w412:sgl, "X值"=w411:sgl, "温度"=w410:sgl, "湿度"=w409:sgl)  [unwired: 2 out]
            n134 = global read "VAR总磷总氮全局变量.vi" "序列号"() -> (w400:string)
            n135 = Bundle By Name(cluster=w397, "时间标识"=w407, "监测值"=w406, "数据标识"=w405, "测量模式"=w398, "单位"=w421, "因子编码"=w420, "标样参考值"=w404, "F0"=w419, "F1"=w418, "F2"=w417, "F3"=w416, "F4"=w415, "F5"=w414, "F6"=w413, "F7"=w412, "X"=w411, "温度"=w410, "湿度"=w409, "量程标识"=w401, "SN"=w400, "数据标记表"=w399, "跨度值"=w395) -> (w393:T1)
            n136 = global read "VAR总磷总氮全局变量.vi" "亚硝氮关键参数"() -> (w389:T9)
            n137 = call "总磷氨氮插入数据.vi"("table"=w392, "关键参数"=w389, "data"=w393) -> ()  [unwired: 12 in, 1 out]
          }
          frame 7 {
            n138 = global read "总磷总氮断电保存全局变量.vi" "质控参数设置"() -> (w463:T8)
            n139 = And(x=w456, y=u16 255) -> (x .and. y?=w469:u16)
            n140 = case shown="\"加标回收\"" w475 {
              tunnel: w461 -> [w495 w502 w509 w516 w521]
              tunnel: [w494 w501 w508 w515 w520] -> w474
              tunnel: [w493 w500 w507 w514 w519] -> w473
              tunnel: [w492 w499 w506 w513 w518] -> w472
              tunnel: [T3."水样测试" ("测量模式") w496 T3."跨度核查" ("测量模式") T3."零点核查" ("测量模式") T3."加标回收" ("测量模式")] -> w465
              tunnel: w463 -> [_ w498 w504 w511 _]
              tunnel: [_ w497 w503 w510 _] -> w471
              tunnel: w459 -> [_ w496 _ _ _]
              tunnel: w458 -> [_ _ _ _ _]
              frame "水样测试", Default {
                n141 = Unbundle By Name(w495) -> ("水样数据时间"=w494:timestamp, "水样实测值"=w493:sgl, "水样数据标识"=w492:string)
              }
              frame "标样核查" {
                n142 = Unbundle By Name(w502) -> ("标样数据时间"=w501:timestamp, "标样实测值"=w500:sgl, "标样数据标识"=w499:string)
                n143 = Unbundle By Name(w498) -> ("硅酸盐标准液标准浓度"=w497:dbl)
              }
              frame "跨度核查" {
                n144 = Unbundle By Name(w509) -> ("跨度核查数据时间"=w508:timestamp, "跨度核查实测值"=w507:sgl, "跨度核查数据标识"=w506:string)
                n145 = Unbundle By Name(w504) -> ("硅酸盐跨度标准液浓度"=w503:dbl)
              }
              frame "零点核查" {
                n146 = Unbundle By Name(w516) -> ("零点核查数据时间"=w515:timestamp, "零点核查实测值"=w514:sgl, "零点核查数据标识"=w513:string)
                n147 = Unbundle By Name(w511) -> ("硅酸盐零点标准液浓度"=w510:dbl)
              }
              frame "加标回收" {
                n148 = Unbundle By Name(w521) -> ("加标回收数据时间"=w520:timestamp, "加标回收实测值"=w519:sgl, "加标回收数据标识"=w518:string)
              }
            }
            n149 = Unbundle By Name(w463) -> ("硅酸盐跨度值"=w462:dbl)
            n150 = case shown="0, 默认" w469 {
              tunnel: ["低量程" ("格式字符串") "高量程" ("格式字符串")] -> w468
              frame 0, Default {
              }
              frame 1 {
              }
            }
            n151 = Unbundle By Name(w461) -> ("单位"=w488:u16, "因子编码"=w487:u32, "F0"=w486:sgl, "F1"=w485:sgl, "F2"=w484:sgl, "F3"=w483:sgl, "F4"=w482:sgl, "F5"=w481:sgl, "F6"=w480:sgl, "F7"=w479:sgl, "X值"=w478:sgl, "温度"=w477:sgl, "湿度"=w476:sgl)  [unwired: 2 out]
            n152 = global read "VAR总磷总氮全局变量.vi" "序列号"() -> (w467:string)
            n153 = Bundle By Name(cluster=w464, "时间标识"=w474, "监测值"=w473, "数据标识"=w472, "测量模式"=w465, "单位"=w488, "因子编码"=w487, "标样参考值"=w471, "F0"=w486, "F1"=w485, "F2"=w484, "F3"=w483, "F4"=w482, "F5"=w481, "F6"=w480, "F7"=w479, "X"=w478, "温度"=w477, "湿度"=w476, "量程标识"=w468, "SN"=w467, "数据标记表"=w466, "跨度值"=w462) -> (w455:T1)
            n154 = global read "VAR总磷总氮全局变量.vi" "硅酸盐关键参数"() -> (w457:T9)
            n155 = call "总磷氨氮插入数据.vi"("table"=w460, "关键参数"=w457, "data"=w455) -> ()  [unwired: 12 in, 1 out]
          }
          frame 8 {
            n156 = global read "总磷总氮断电保存全局变量.vi" "质控参数设置"() -> (w530:T8)
            n157 = And(x=w522, y=u16 255) -> (x .and. y?=w536:u16)
            n158 = case shown="\"加标回收\"" w542 {
              tunnel: w528 -> [w562 w569 w576 w583 w588]
              tunnel: [w561 w568 w575 w582 w587] -> w541
              tunnel: [w560 w567 w574 w581 w586] -> w540
              tunnel: [w559 w566 w573 w580 w585] -> w539
              tunnel: [T3."水样测试" ("测量模式") w563 T3."跨度核查" ("测量模式") T3."零点核查" ("测量模式") T3."加标回收" ("测量模式")] -> w532
              tunnel: w530 -> [_ w565 w571 w578 _]
              tunnel: [_ w564 w570 w577 _] -> w538
              tunnel: w525 -> [_ _ _ _ _]
              tunnel: w524 -> [_ w563 _ _ _]
              frame "水样测试", Default {
                n159 = Unbundle By Name(w562) -> ("水样数据时间"=w561:timestamp, "水样实测值"=w560:sgl, "水样数据标识"=w559:string)
              }
              frame "标样核查" {
                n160 = Unbundle By Name(w569) -> ("标样数据时间"=w568:timestamp, "标样实测值"=w567:sgl, "标样数据标识"=w566:string)
                n161 = Unbundle By Name(w565) -> ("硫化物标准液标准浓度"=w564:dbl)
              }
              frame "跨度核查" {
                n162 = Unbundle By Name(w576) -> ("跨度核查数据时间"=w575:timestamp, "跨度核查实测值"=w574:sgl, "跨度核查数据标识"=w573:string)
                n163 = Unbundle By Name(w571) -> ("硫化物跨度标准液浓度"=w570:dbl)
              }
              frame "零点核查" {
                n164 = Unbundle By Name(w583) -> ("零点核查数据时间"=w582:timestamp, "零点核查实测值"=w581:sgl, "零点核查数据标识"=w580:string)
                n165 = Unbundle By Name(w578) -> ("硫化物零点标准液浓度"=w577:dbl)
              }
              frame "加标回收" {
                n166 = Unbundle By Name(w588) -> ("加标回收数据时间"=w587:timestamp, "加标回收实测值"=w586:sgl, "加标回收数据标识"=w585:string)
              }
            }
            n167 = Unbundle By Name(w530) -> ("硫化物跨度值"=w529:dbl)
            n168 = case shown="0, 默认" w536 {
              tunnel: ["低量程" ("格式字符串") "高量程" ("格式字符串")] -> w535
              frame 0, Default {
              }
              frame 1 {
              }
            }
            n169 = Unbundle By Name(w528) -> ("单位"=w555:u16, "因子编码"=w554:u32, "F0"=w553:sgl, "F1"=w552:sgl, "F2"=w551:sgl, "F3"=w550:sgl, "F4"=w549:sgl, "F5"=w548:sgl, "F6"=w547:sgl, "F7"=w546:sgl, "X值"=w545:sgl, "温度"=w544:sgl, "湿度"=w543:sgl)  [unwired: 2 out]
            n170 = global read "VAR总磷总氮全局变量.vi" "序列号"() -> (w534:string)
            n171 = Bundle By Name(cluster=w531, "时间标识"=w541, "监测值"=w540, "数据标识"=w539, "测量模式"=w532, "单位"=w555, "因子编码"=w554, "标样参考值"=w538, "F0"=w553, "F1"=w552, "F2"=w551, "F3"=w550, "F4"=w549, "F5"=w548, "F6"=w547, "F7"=w546, "X"=w545, "温度"=w544, "湿度"=w543, "量程标识"=w535, "SN"=w534, "数据标记表"=w533, "跨度值"=w529) -> (w527:T1)
            n172 = global read "VAR总磷总氮全局变量.vi" "硫化物关键参数"() -> (w523:T9)
            n173 = call "总磷氨氮插入数据.vi"("table"=w526, "关键参数"=w523, "data"=w527) -> ()  [unwired: 12 in, 1 out]
          }
          frame 22 {
            n174 = global read "总磷总氮断电保存全局变量.vi" "质控参数设置"() -> (w596:T8)
            n175 = And(x=w589, y=u16 255) -> (x .and. y?=w603:u16)
            n176 = case shown="\"加标回收\"" w609 {
              tunnel: w594 -> [w629 w636 w643 w650 w655]
              tunnel: [w628 w635 w642 w649 w654] -> w608
              tunnel: [w627 w634 w641 w648 w653] -> w607
              tunnel: [w626 w633 w640 w647 w652] -> w606
              tunnel: [T3."水样测试" ("测量模式") w630 T3."跨度核查" ("测量模式") T3."零点核查" ("测量模式") T3."加标回收" ("测量模式")] -> w599
              tunnel: w596 -> [_ w632 w638 w645 _]
              tunnel: [_ w631 w637 w644 _] -> w605
              tunnel: w592 -> [_ _ _ _ _]
              tunnel: w591 -> [_ w630 _ _ _]
              frame "水样测试", Default {
                n177 = Unbundle By Name(w629) -> ("水样数据时间"=w628:timestamp, "水样实测值"=w627:sgl, "水样数据标识"=w626:string)
              }
              frame "标样核查" {
                n178 = Unbundle By Name(w636) -> ("标样数据时间"=w635:timestamp, "标样实测值"=w634:sgl, "标样数据标识"=w633:string)
                n179 = Unbundle By Name(w632) -> ("COD标准液标准浓度"=w631:dbl)
              }
              frame "跨度核查" {
                n180 = Unbundle By Name(w643) -> ("跨度核查数据时间"=w642:timestamp, "跨度核查实测值"=w641:sgl, "跨度核查数据标识"=w640:string)
                n181 = Unbundle By Name(w638) -> ("COD跨度标准液浓度"=w637:dbl)
              }
              frame "零点核查" {
                n182 = Unbundle By Name(w650) -> ("零点核查数据时间"=w649:timestamp, "零点核查实测值"=w648:sgl, "零点核查数据标识"=w647:string)
                n183 = Unbundle By Name(w645) -> ("COD零点标准液浓度"=w644:dbl)
              }
              frame "加标回收" {
                n184 = Unbundle By Name(w655) -> ("加标回收数据时间"=w654:timestamp, "加标回收实测值"=w653:sgl, "加标回收数据标识"=w652:string)
              }
            }
            n185 = Unbundle By Name(w596) -> ("COD跨度值"=w595:dbl)
            n186 = case shown="0, 默认" w603 {
              tunnel: ["低量程" ("格式字符串") "高量程" ("格式字符串")] -> w602
              frame 0, Default {
              }
              frame 1 {
              }
            }
            n187 = Unbundle By Name(w594) -> ("单位"=w622:u16, "因子编码"=w621:u32, "F0"=w620:sgl, "F1"=w619:sgl, "F2"=w618:sgl, "F3"=w617:sgl, "F4"=w616:sgl, "F5"=w615:sgl, "F6"=w614:sgl, "F7"=w613:sgl, "X值"=w612:sgl, "温度"=w611:sgl, "湿度"=w610:sgl)  [unwired: 2 out]
            n188 = global read "VAR总磷总氮全局变量.vi" "序列号"() -> (w601:string)
            n189 = Bundle By Name(cluster=w598, "时间标识"=w608, "监测值"=w607, "数据标识"=w606, "测量模式"=w599, "单位"=w622, "因子编码"=w621, "标样参考值"=w605, "F0"=w620, "F1"=w619, "F2"=w618, "F3"=w617, "F4"=w616, "F5"=w615, "F6"=w614, "F7"=w613, "X"=w612, "温度"=w611, "湿度"=w610, "量程标识"=w602, "SN"=w601, "数据标记表"=w600, "跨度值"=w595) -> (w597:T1)
            n190 = global read "VAR总磷总氮全局变量.vi" "CODcr关键参数"() -> (w590:T9)
            n191 = call "总磷氨氮插入数据.vi"("table"=w593, "关键参数"=w590, "data"=w597) -> ()  [unwired: 12 in, 1 out]
          }
        }
      }
    }
  }
